vi "Keithley2612b_IV_vg_vd.vi"(3 "Error Query (False)":bool, 4 "Limit":dbl=1.0, 7 "Source Function (Current)":enum32{"Current", "Voltage"}(ring)=enum."Voltage", 8 "error in (no error)":errorcluster, 9 "Channel (Channel A)":T1, 10 "Node (0-64)":i8 min=0 max=64 step=1, 11 "VISA resource name":refnum<visa-resource-name>) -> (0 "error out":errorcluster)   [LabVIEW 2016]
doc: "This example shows how to configure the source and take a measurement."
uses:
  <instrlib>/Keithley 2600 Series/Public/Channel.ctl
  <vilib>/express/express shared/transition.llb/Dynamic To Waveform Array.vi
  <vilib>/express/express signal manip/GetorSetDDTAttributes/Set DDT Attributes/SetT0.vi
  <vilib>/express/express shared/transition.llb/Waveform Array To Dynamic.vi
  <vilib>/express/express signal manip/GetorSetDDTAttributes/Set DDT Attributes/Set DDT Properties.xnode
  <instrlib>/Keithley 2600 Series/Keithley 2600 Series.lvlib
panel:
  in  "Delay (s) 2":dbl
  in  "Step Size 2":dbl
  in  "End Voltage 2":dbl
  in  "Start Voltage 2":dbl
  in  "Limit 2":dbl=1.0
  out "Current Output 2":string
  out "Voltage Output 2":string
  out "Current Number Past 2":dbl
  in  "Source Function (Current) 2":enum32{"Current", "Voltage"}(ring)=enum."Voltage"
  in  "Channel (Channel A) 2":T1
  out "Current Number Past":dbl
  out "Voltage Output":string
  out "Current Output":string
  in  "Delay (s)":dbl
  in  "Step Size":dbl
  in  "End Voltage":dbl
  in  "Start Voltage":dbl
  # "(c) 2008 Keithley Instruments, Inc.  ALL RIGHTS RESERVED."
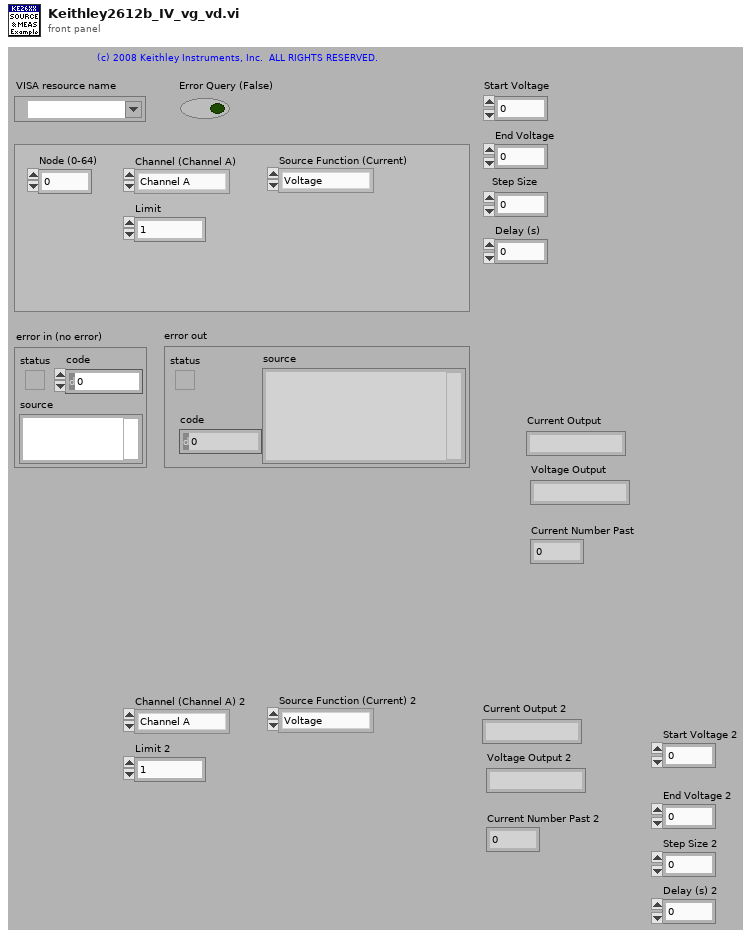
[diagram p1: front panel]
types:
  T1 = typedef "Keithley 2600 Series.lvlib/Channel.ctl" = enum32{"Channel A", "Channel B"}
  T2 = typedef "NI_Matrix.lvlib/RealMatrix.ctl" = dbl[][]
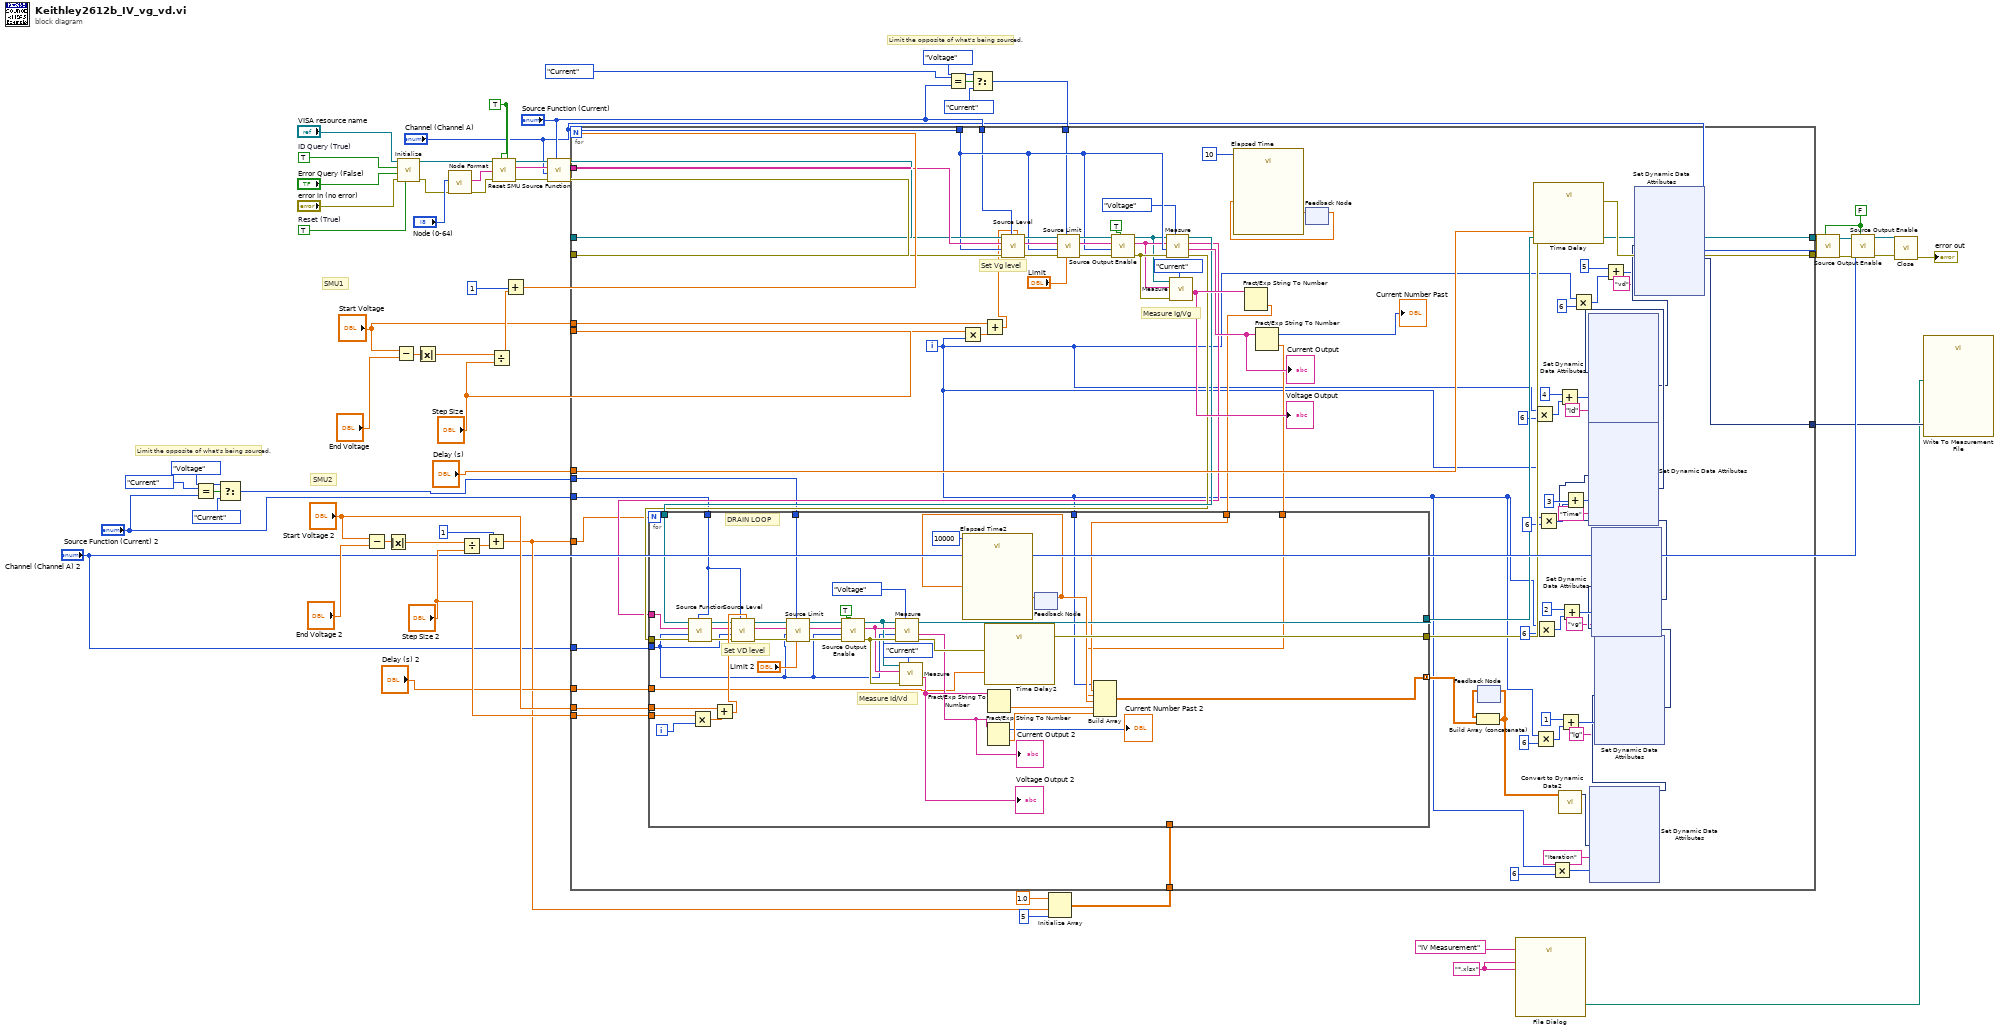
[diagram p0: block diagram]
diagram:
  w15 = "*.xlsx"
  w29 = TRUE
  w5 = FALSE ("Output (Off)")
  w61 = TRUE  # Reset (True)
  w64 = TRUE  # ID Query (True)
  # "SMU2"
  # "SMU1"
  # "Limit the opposite of what's being sourced."
  # "Limit the opposite of what's being sourced."
  n1 = Equal?(x=enum32{"Current", "Voltage"}."Current", y="Source Function (Current) 2") -> (x = y?=w35:bool)
  n2 = Select(t=enum32{"Current", "Voltage"}."Voltage" ("x"), s=w35, f=enum32{"Current", "Voltage"}."Current") -> (s? t:f=w16:enum32{"Current", "Voltage"})
  n3 = Subtract(x="Start Voltage 2", y="End Voltage 2") -> (x-y=w24:dbl)
  n4 = Absolute Value(x=w24) -> (abs(x)=w23:dbl)
  n5 = Subtract(x="Start Voltage", y="End Voltage") -> (x-y=w44:dbl)
  n6 = call <instrlib>:"Initialize.vi"("Reset (True)"=w61, "error in (no error)"="error in (no error)", "Error Query (False)"="Error Query (False)", "ID Query (True)"=w64, "VISA resource name"="VISA resource name") -> ("error out"=w37:errorcluster, "VISA resource name out"=w30:refnum<visa-resource-name>)  [unwired: 1 in, 4 out]
  n7 = Absolute Value(x=w44) -> (abs(x)=w43:dbl)
  n8 = call <instrlib>:"Node Format.vi"("error in"=w37, "Node (0-64)"="Node (0-64)") -> ("error out"=w57:errorcluster, "Formatted Node"=w58:string)  [unwired: 8 out]
  n9 = Divide(x=w23, y="Step Size 2") -> (x/y=w21:dbl)
  n10 = Add(x=1, y=w21) -> (x+y=w10:dbl)
  n11 = Divide(x=w43, y="Step Size") -> (x/y=w41:dbl)
  n12 = call <instrlib>:"Reset SMU.vi"("SMU B (No)"=w29, "SMU A (No)"=w29, "error in (no error)"=w57, "Node In"=w58, "VISA resource name"=w30) -> ("error out"=w28:errorcluster, "Node Out"=w26:string, "VISA resource name out"=w27:refnum<visa-resource-name>)  [unwired: 4 out]
  n13 = Add(x=1, y=w41) -> (x+y=w40:dbl)
  n14 = call <instrlib>:"Source Function.vi"("Function (Current)"="Source Function (Current)", "error in (no error)"=w28, "Channel (Channel A)"="Channel (Channel A)", "Node In"=w26, "VISA resource name"=w27) -> ("error out"=w55:errorcluster, "Node Out"=w54:string, "VISA resource name out"=w53:refnum<visa-resource-name>)  [unwired: 4 out]
  n15 = Equal?(x=enum32{"Current", "Voltage"}."Current", y="Source Function (Current)") -> (x = y?=w59:bool)
  n16 = Select(t=enum32{"Current", "Voltage"}."Voltage" ("x"), s=w59, f=enum32{"Current", "Voltage"}."Current") -> (s? t:f=w47:enum32{"Current", "Voltage"})
  n17 = Initialize Array(1.0, w10, 5) -> (w11:dbl[][])
  n18 = for {
    N: w40 -> [_]
    tunnel: w55 -> [w141]
    tunnel: w54 -> [w140]
    tunnel: w53 -> [w139]
    tunnel: "Channel (Channel A)" -> [w138]
    tunnel: "Source Function (Current)" -> [w135]
    tunnel: "Step Size" -> [w131]
    tunnel: "Start Voltage" -> [w136]
    tunnel: w47 -> [w134]
    tunnel: [w111] -> w8
    tunnel: [w132] -> w7
    tunnel: "Delay (s)" -> [w133]
    tunnel: "Step Size 2" -> [w115]
    tunnel: "Start Voltage 2" -> [w114]
    tunnel: w10 -> [w113]
    tunnel: "Delay (s) 2" -> [w110]
    tunnel: "Channel (Channel A) 2" -> [w109]
    tunnel: "Source Function (Current) 2" -> [w108]
    tunnel: w16 -> [w107]
    tunnel: w11 -> [w104]
    tunnel: [w65] -> w2
    i -> [w66]
    # "Measure Ig/Vg"
    # "Set Vg level"
    n19 = Multiply(x=w131, y=w66) -> (x*y=w137:dbl)
    n20 = Add(x=w136, y=w137) -> (x+y=w119:dbl)
    n21 = call <instrlib>:"Source Level.vi"("Level (0.000)"=w119, "Function (Current)"=w135, "error in (no error)"=w141, "Channel (Channel A)"=w138, "Node In"=w140, "VISA resource name"=w139) -> ("error out"=w142:errorcluster, "Node Out"=w147:string, "VISA resource name out"=w143:refnum<visa-resource-name>)  [unwired: 3 out]
    n22 = call <instrlib>:"Source Limit.vi"("Limit (0.000)"="Limit", "Function (Current)"=w134, "error in (no error)"=w142, "Channel (Channel A)"=w138, "Node In"=w147, "VISA resource name"=w143) -> ("error out"=w145:errorcluster, "Node Out"=w148:string, "VISA resource name out"=w144:refnum<visa-resource-name>)  [unwired: 3 out]
    n23 = call <instrlib>:"Source Output Enable.vi"("Output (Off)"=TRUE, "error in (no error)"=w145, "Channel (Channel A)"=w138, "Node In"=w148, "VISA resource name"=w144) -> ("error out"=w129:errorcluster, "Node Out"=w128:string, "VISA resource name out"=w127:refnum<visa-resource-name>)  [unwired: 4 out]
    n24 = call <instrlib>:"Measure.vi"("Function (Current)"=enum32{"Current", "Voltage"}."Voltage" ("x"), "error in (no error)"=w129, "Channel (Channel A)"=w138, "Node In"=w128, "VISA resource name"=w127) -> ("error out"=w117:errorcluster, "Output"=w123:string, "Node Out"=w116:string, "VISA resource name out"=w118:refnum<visa-resource-name>)  [unwired: 2 in, 1 out]
    "Current Output" <- w123
    n25 = call <instrlib>:"Measure.vi"("Function (Current)"=enum32{"Current", "Voltage"}."Current" ("x"), "error in (no error)"=w129, "Node In"=w128, "VISA resource name"=w127) -> ("Output"=w124:string)  [unwired: 3 in, 4 out]
    "Voltage Output" <- w124
    n26 = Fract/Exp String To Number(string=w124) -> (number=w106:dbl)  [unwired: 3 in, 1 out]
    n27 = Fract/Exp String To Number(string=w123) -> (offset past number=→"Current Number Past":i32, number=w105:dbl)  [unwired: 3 in]
    n28 = for {
      N: w113 -> [_]
      tunnel: w116 -> [w238]
      tunnel: w115 -> [w257]
      tunnel: w114 -> [w261]
      tunnel: w107 -> [w260]
      tunnel: [w242] -> w111
      tunnel: [w258] -> w112
      tunnel: w117 -> [w239]
      tunnel: w118 -> [w237]
      tunnel: w110 -> [w241]
      tunnel: w109 -> [w234]
      tunnel: w108 -> [w231]
      tunnel: w106 -> [w233]
      tunnel: w105 -> [w232]
      tunnel: w104 -> [_]
      tunnel: [w229] -> w102 mode=concatenating
      tunnel: w66 -> [w228]
      i -> [w230]
      # "Set VD level"
      # "Measure Id/Vd"
      # "DRAIN LOOP"
      n29 = call <instrlib>:"Source Function.vi"("Function (Current)"=w231, "error in (no error)"=w239, "Channel (Channel A)"=w234, "Node In"=w238, "VISA resource name"=w237) -> ("error out"=w240:errorcluster, "Node Out"=w236:string, "VISA resource name out"=w235:refnum<visa-resource-name>)  [unwired: 4 out]
      n30 = Multiply(x=w257, y=w230) -> (x*y=w262:dbl)
      n31 = Add(x=w261, y=w262) -> (x+y=w243:dbl)
      n32 = call <instrlib>:"Source Level.vi"("Level (0.000)"=w243, "Function (Current)"=w231, "error in (no error)"=w240, "Channel (Channel A)"=w234, "Node In"=w236, "VISA resource name"=w235) -> ("error out"=w263:errorcluster, "Node Out"=w268:string, "VISA resource name out"=w264:refnum<visa-resource-name>)  [unwired: 3 out]
      n33 = call <instrlib>:"Source Limit.vi"("Limit (0.000)"="Limit 2", "Function (Current)"=w260, "error in (no error)"=w263, "Channel (Channel A)"=w234, "Node In"=w268, "VISA resource name"=w264) -> ("error out"=w266:errorcluster, "Node Out"=w269:string, "VISA resource name out"=w265:refnum<visa-resource-name>)  [unwired: 3 out]
      n34 = call <instrlib>:"Source Output Enable.vi"("Output (Off)"=TRUE, "error in (no error)"=w266, "Channel (Channel A)"=w234, "Node In"=w269, "VISA resource name"=w265) -> ("error out"=w255:errorcluster, "Node Out"=w254:string, "VISA resource name out"=w253:refnum<visa-resource-name>)  [unwired: 4 out]
      n35 = call <instrlib>:"Measure.vi"("Function (Current)"=enum32{"Current", "Voltage"}."Voltage" ("x"), "error in (no error)"=w255, "Channel (Channel A)"=w234, "Node In"=w254, "VISA resource name"=w253) -> ("error out"=w259:errorcluster, "Output"=w248:string, "VISA resource name out"=w242:refnum<visa-resource-name>)  [unwired: 2 in, 2 out]
      "Current Output 2" <- w248
      n36 = call <instrlib>:"Measure.vi"("Function (Current)"=enum32{"Current", "Voltage"}."Current" ("x"), "error in (no error)"=w255, "Node In"=w254, "VISA resource name"=w253) -> ("Output"=w250:string)  [unwired: 3 in, 4 out]
      "Voltage Output 2" <- w250
      n37 = call "Time Delay2"("error in (no error)"=w259, "Delay Time (s)"=w241) -> ("error out"=w258:errorcluster)  [unwired: 9 in]
      n38 = Fract/Exp String To Number(string=w248) -> (offset past number=→"Current Number Past 2":i32, number=w247:dbl)  [unwired: 3 in]
      n39 = Fract/Exp String To Number(string=w250) -> (number=w249:dbl)  [unwired: 3 in, 1 out]
      n40 = feedback #1() -> (w244:dbl)  [unwired: 1 in]
      n41 = call "Elapsed Time2"("Time Target (s)"=10000, "Set Start Time (s)"=w244) -> ("Elapsed Time (s)"=w251:dbl)  [unwired: 10 in, 7 out]
      n42 = feedback-in #1(w251) -> ()
      n43 = Build Array(w228, w233, w232, w244, w249, w247) -> (w229:T2)
    }
    n44 = feedback #2() -> (w120:dbl)  [unwired: 1 in]
    n45 = call "Elapsed Time"("Time Target (s)"=10, "Set Start Time (s)"=w120) -> ("Elapsed Time (s)"=w125:dbl)  [unwired: 10 in, 7 out]
    n46 = feedback-in #2(w125) -> ()
    n47 = feedback #3() -> (w103:T2)  [unwired: 1 in]
    n48 = Build Array (concatenate)(w103, w102) -> (w83:T2)
    n49 = feedback-in #3(w83) -> ()
    n50 = Multiply(x=w66, y=6) -> (x*y=w86:i32)
    n51 = call "Time Delay"("error in (no error)"=w112, "Delay Time (s)"=w133) -> ("error out"=w132:errorcluster)  [unwired: 9 in]
    n52 = Multiply(x=w66, y=6) -> (x*y=w98:i32)
    n53 = Multiply(x=w66, y=6) -> (x*y=w94:i32)
    n54 = Multiply(x=w66, y=6) -> (x*y=w90:i32)
    n55 = Multiply(x=w66, y=6) -> (x*y=w100:i32)
    n56 = Add(x=4, y=w86) -> (x+y=w84:i32)
    n57 = call "Convert to Dynamic Data2"("2D Array"=w83) -> ("Dynamic Data Type"=w82:dynamicdata)  [unwired: 3 in]
    n58 = Add(x=1, y=w98) -> (x+y=w96:i32)
    n59 = Add(x=2, y=w94) -> (x+y=w92:i32)
    n60 = Add(x=3, y=w90) -> (x+y=w88:i32)
    n61 = Multiply(x=w66, y=6) -> (x*y=w69:i32)
    n62 = xnode "Set Dynamic Data Attributes"("Signals In"=w82, "Signal Name"="Iteration", "Signal Index"=w100) -> ("Signals Out"=w81:dynamicdata)  [unwired: 1 in, 1 out]
    n63 = xnode "Set Dynamic Data Attributes"("Signals In"=w81, "Signal Index"=w96, "Signal Name"="ig") -> ("Signals Out"=w80:dynamicdata)  [unwired: 1 in, 1 out]
    n64 = xnode "Set Dynamic Data Attributes"("Signals In"=w80, "Signal Index"=w92, "Signal Name"="vg") -> ("Signals Out"=w79:dynamicdata)  [unwired: 1 in, 1 out]
    n65 = xnode "Set Dynamic Data Attributes"("Signals In"=w79, "Signal Index"=w88, "Signal Name"="Time") -> ("Signals Out"=w78:dynamicdata)  [unwired: 1 in, 1 out]
    n66 = xnode "Set Dynamic Data Attributes"("Signals In"=w78, "Signal Index"=w84, "Signal Name"="id") -> ("Signals Out"=w73:dynamicdata)  [unwired: 1 in, 1 out]
    n67 = Add(x=5, y=w69) -> (x+y=w68:i32)
    n68 = xnode "Set Dynamic Data Attributes"("Signals In"=w73, "Signal Index"=w68, "Signal Name"="vd") -> ("Signals Out"=w65:dynamicdata)  [unwired: 1 in, 1 out]
  }
  n69 = call "File Dialog"("default name"="IV Measurement", "pattern (all files)"=w15, "pattern label"=w15) -> ("selected path"=w1:path)  [unwired: 9 in, 3 out]
  n70 = call <instrlib>:"Source Output Enable.vi"("Output (Off)"=w5, "error in (no error)"=w7, "Channel (Channel A)"="Channel (Channel A)", "VISA resource name"=w8) -> ("error out"=w6:errorcluster, "VISA resource name out"=w9:refnum<visa-resource-name>)  [unwired: 1 in, 5 out]
  n71 = call <instrlib>:"Source Output Enable.vi"("Output (Off)"=w5, "error in (no error)"=w6, "Channel (Channel A)"="Channel (Channel A) 2", "VISA resource name"=w9) -> ("error out"=w48:errorcluster, "VISA resource name out"=w49:refnum<visa-resource-name>)  [unwired: 1 in, 5 out]
  n72 = call <instrlib>:"Close.vi"("error in (no error)"=w48, "VISA resource name"=w49) -> ("error out"=→"error out":errorcluster)  [unwired: 9 out]
  n73 = call "Write To Measurement File"("Signals"=w2, "Filename"=w1) -> ()  [unwired: 15 in, 3 out]
